vi "Init Teststand.vi"(8 "error in (no error)":errorcluster, 10 "Sequence Context In":refnum<k7>, 11 "Teststand in":refnum<class "Teststand.lvclass">) -> (0 "error out":errorcluster, 3 "Teststand out":refnum<class "Teststand.lvclass">)   [LabVIEW 2023, in "HardwareAbstractionLayer_LVOOP.lvlib" / "Teststand.lvclass"]
doc: "This vi is used to Teststand init reference and termination."
uses:
  Teststand.lvclass
  Teststand.lvclass/Teststand.ctl
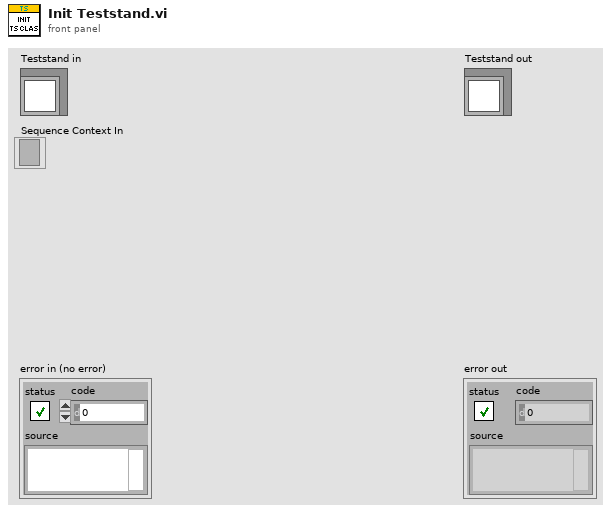
[diagram p1: front panel]
types:
  T1 = typedef "TestStand - Status Monitor.ctl" = cluster{"Sequence Context":refnum<k7>, "Execution":refnum<k7>, "Termination Monitor":refnum<k7>}
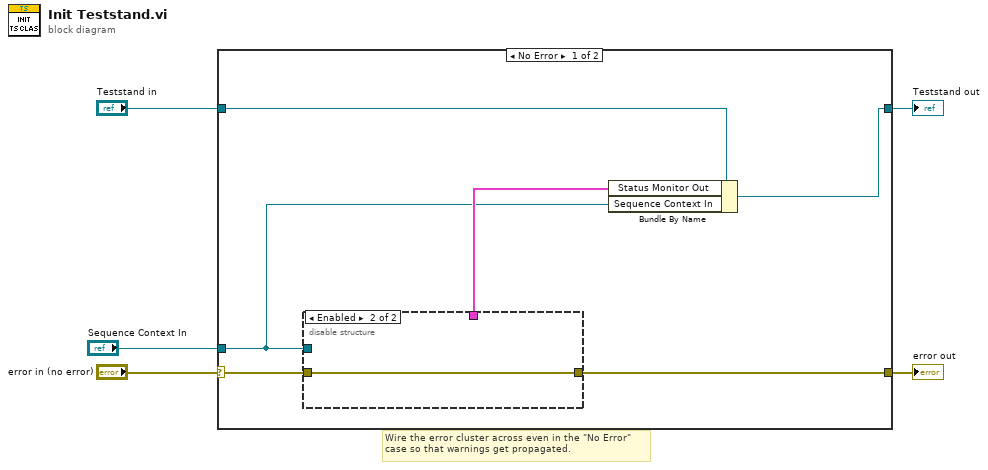
[diagram p0: block diagram]
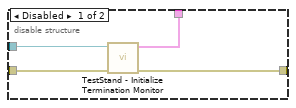
[diagram p2: hidden frame]
diagram:
  # "Wire the error cluster across even in the \"No Error\"\ncase so that warnings get propagated."
  n1 = case shown="No Error" "error in (no error)" {
    selector: "error in (no error)" -> [w11 w18]
    tunnel: [w7 w18] -> w4
    tunnel: [w6 w17] -> w2
    tunnel: "Teststand in" -> [w10 w17]
    tunnel: "Sequence Context In" -> [w8 _]
    frame No Error {
      n2 = disable-structure shown="Enabled" {
        disable-tunnel: w11 -> [w15 w16]
        disable-tunnel: [w14 _] -> w9
        disable-tunnel: w8 -> [w13 _]
        disable-tunnel: [w12 w16] -> w7
        frame Disabled {
          n3 = call <vilib>:"TestStand - Initialize Termination Monitor.vi"("error in (no error)"=w15, "Sequence Context In"=w13) -> ("error out"=w12:errorcluster, "Status Monitor Out"=w14:T1)  [unwired: 8 in]
        }
        frame Enabled {
        }
      }
      n4 = Bundle By Name(cluster=w10, "Status Monitor Out"=w9, "Sequence Context In"=w8) -> (w6:refnum<class "Teststand.lvclass">)
    }
    frame Error {
    }
  }
  "error out" <- w4
  "Teststand out" <- w2
